vi "Set-to-startup-condition.vi"(8 "error in (no error)":errorcluster, 11 "Panes in":T1) -> (0 "error out":errorcluster, 3 "Panes out":T1)   [LabVIEW 2013, in "MaterialCharacterization.lvlib" / "MC-UI.lvclass"]
uses:
  MC-UI.lvclass
  Panes-reference.ctl
  MC-UI.lvclass/MC-UI.ctl
  Read-Panes.vi
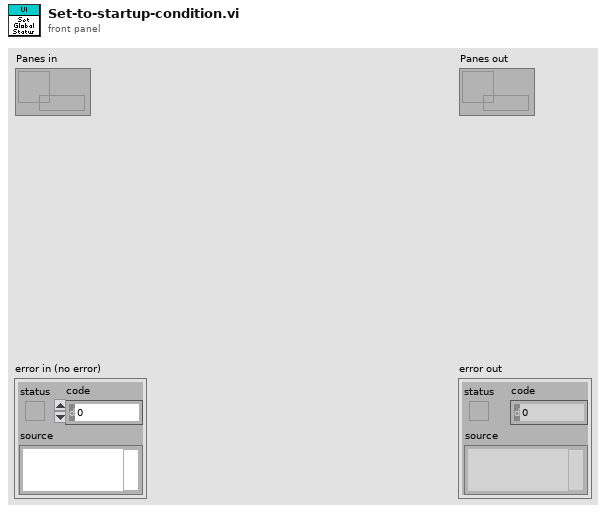
[diagram p1: front panel]
types:
  T1 = typedef "MaterialCharacterization.lvlib/MC-UI.lvclass/Panes-reference.ctl" = refnum<data-value>
  T2 = typedef "TemplateProject.lvlib/TP-UI.lvclass/Pane-settings.ctl" = cluster{"Pane-name":T3, "Startup status":bool, "Current status":bool, "Splitters":T4[], "Pane-reference":refnum<vi>}
  T3 = typedef "TemplateProject.lvlib/TP-UI.lvclass/Pane-names.ctl" = enum16{"Toolbar", "Help bar", "Toolbar lower border", "Center panel", "Main panel", "Settings panel", "Status bar upper border", "General state bar", "Information bar"}
  T4 = typedef "TemplateProject.lvlib/TP-UI.lvclass/Splitter-settings.ctl" = cluster{"Splitter-name":T5, "Position shown":i32, "Position hidden":i32, "Splitter reference":refnum<vi>}
  T5 = typedef "TemplateProject.lvlib/TP-UI.lvclass/Splitter-names.ctl" = enum16{"Upper toolbar splitter", "Help bar splitter", "Lower toolbar splitter", "Upper status bar splitter", "Lower status bar splitter", "Left status bar splitter", "Settings splitter"}
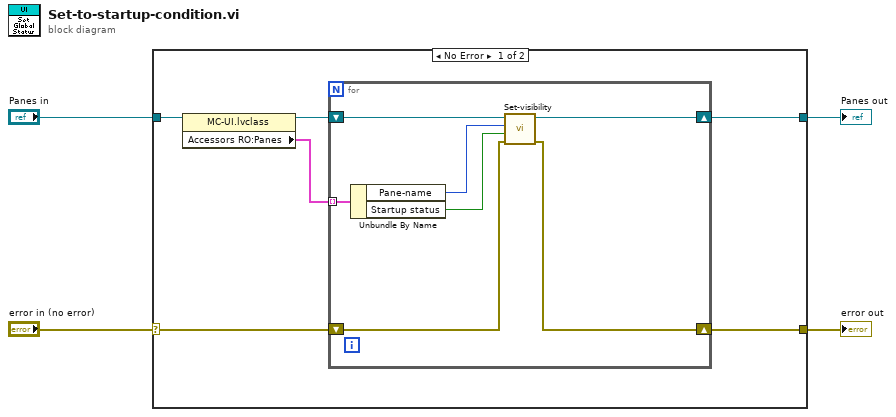
[diagram p0: block diagram]
diagram:
  n1 = case shown="No Error" "error in (no error)" {
    selector: "error in (no error)" -> [w7 w18]
    tunnel: [w5 w18] -> w3
    tunnel: [w6 w19] -> w1
    tunnel: "Panes in" -> [w10 w19]
    frame No Error {
      n2 = property class="MC-UI.lvclass"(reference=w10) -> (reference out=w9:T1, "Accessors RO:Panes"=w8:T2[])  [unwired: 1 in, 1 out]
      n3 = for {
        shift-right: [w11] -> w6
        shift-left: w9 -> [w16]
        tunnel: w8 -> [w17] mode=indexing
        shift-right: [w12] -> w5
        shift-left: w7 -> [w13]
        n4 = Unbundle By Name(w17) -> ("Pane-name"=w15:T3, "Startup status"=w14:bool)
        n5 = call "Set-visibility.vi"("error in (no error)"=w13, "Visibility"=w14, "Pane"=w15, "Panes in"=w16) -> ("error out"=w12:errorcluster, "Panes out"=w11:T1)  [unwired: 6 in]
      }
    }
    frame Error {
    }
  }
  "error out" <- w3
  "Panes out" <- w1
